vi "display node data.vi"(8 "error in":errorcluster, 11 "CEF_serializable node in":refnum<class "CEF_serializable node.lvclass">) -> (0 "error out":errorcluster, 3 "CEF_serializable node out":refnum<class "CEF_serializable node.lvclass">)   [LabVIEW 2025, in "CEF.lvlib" / "CEF_serializable node.lvclass"]
doc: "Copyright 2017 National Instruments Corporation\n\nLicensed under the Apache License, Version 2.0 (the \"License\"); you may not use this file except in compliance with the License. You may obtain a copy of the License at http://www.apache.org/licenses/LICENSE-2.0\nUnless required by applicable law or agreed to in writing, software distributed under the License is distributed on an \"AS IS\" BASIS, WITHOUT WARRANTIES OR CONDITIONS OF ANY KIND, either express or implied. See the License for the specific language governing permissions and limitations under the License."
uses:
  CEF_serializable node.lvclass
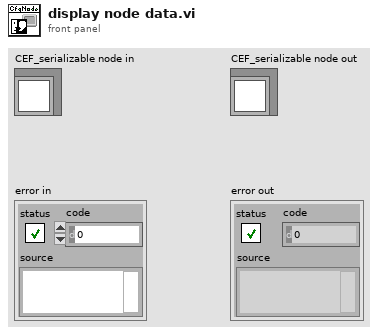
[diagram p1: front panel]
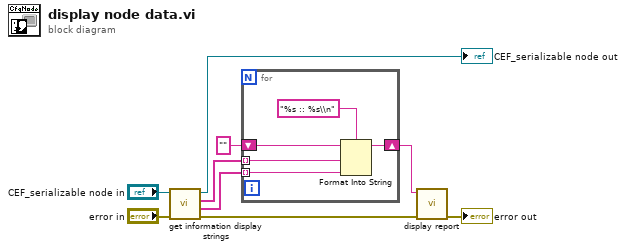
[diagram p0: block diagram]
diagram:
  n1 = call-dynamic "get information display strings.vi"("error in"="error in", "CEF_serializable node in"="CEF_serializable node in") -> ("error out"=w1:errorcluster, "Data"=w5:string[], "Labels"=w6:string[], "CEF_serializable node out"=→"CEF_serializable node out":refnum<class "CEF_serializable node.lvclass">)  [unwired: 6 in]
  n2 = for {
    tunnel: w6 -> [w14] mode=indexing
    tunnel: w5 -> [w13] mode=indexing
    shift-right: [w11] -> w2
    shift-left: "" -> [w10]
    n3 = Format Into String(format string="%s :: %s\\n", initial string=w10, w14, w13) -> (resulting string=w11:string)  [unwired: 1 in, 1 out]
  }
  n4 = call "display report.vi"("error in"=w1, "data to display"=w2) -> ("error out"=→"error out":errorcluster)  [unwired: 9 in]
